vi "Create Live Random Data Tag Array.vi"() -> ()   [LabVIEW 2014]
uses:
  Tag.lvclass
  Anchor/Anchor.lvclass
panel:
  in  "Max h variatie":dbl=30.0 format="%#_13g"
  in  "Max V variatie":dbl=10.0 format="%#_13g"
  in  "DistanceLimitAnchor":dbl=150.0
  in  "Input AnchorArray":refnum<class "Anchor.lvclass">[](array[class])
  out "OutputArray":T1(array[cluster])
  in  "InputArray":T1(array[cluster])
  in  "TagsArray":refnum<class "Tag.lvclass">[](array[class])
  # "This VI creates a number of random data for each assigned tag in its array."
  # "tagID, X, Y, distances"
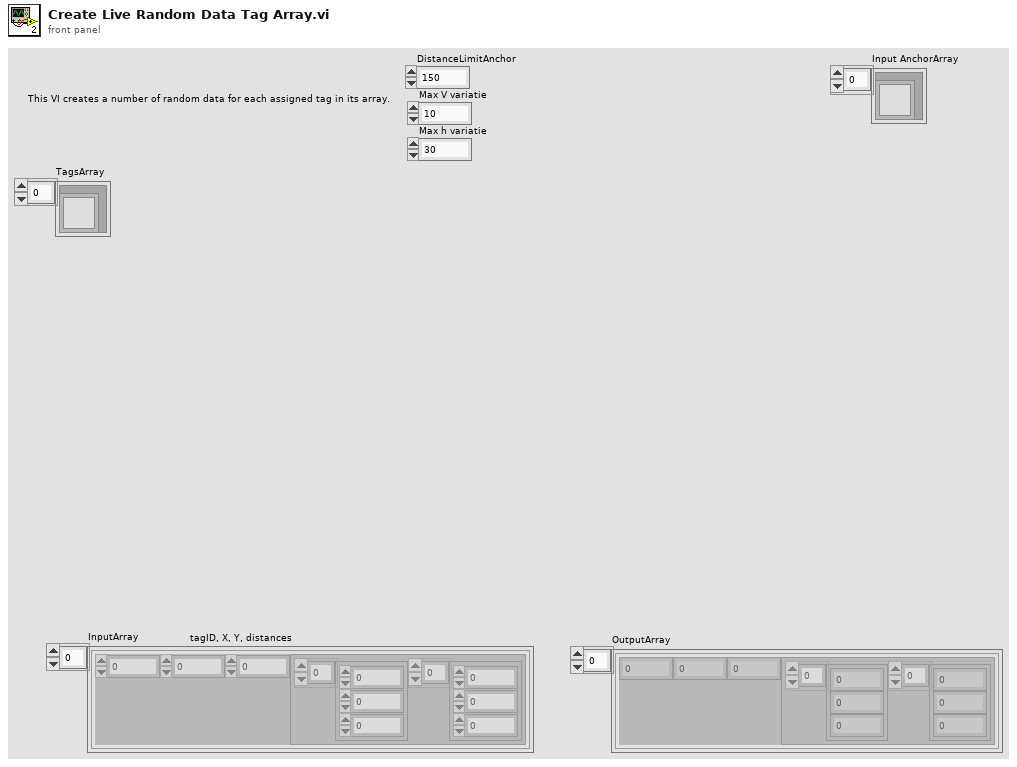
[diagram p1: front panel]
types:
  T1 = cluster{"Tag":dbl, "X":dbl, "Y":dbl, "AnchorIDDistanceCluster":cluster{"AnchorIDArray":dbl[], "AnchorDistancesArray":dbl[]}}[]
  T2 = cluster{"Tag.lvclass":refnum<class "Tag.lvclass">, "Intersections":cluster{"time [ms]":dbl, "x":dbl, "y":dbl, "Fout":bool, "Goed":bool}[]}[]
  T3 = cluster{"time [ms]":dbl, "x":dbl, "y":dbl, "Fout":bool, "Goed":bool}[]
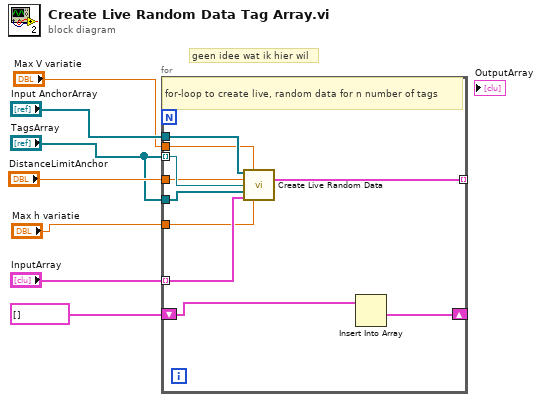
[diagram p0: block diagram]
diagram:
  # "geen idee wat ik hier wil"
  n1 = for {
    tunnel: "TagsArray" -> [w17] mode=indexing
    tunnel: "InputArray" -> [w15] mode=indexing
    tunnel: [w16] -> _ mode=indexing
    shift-right: [w14] -> _
    shift-left: T2 [] -> [w13]
    tunnel: "Input AnchorArray" -> [w12]
    tunnel: "DistanceLimitAnchor" -> [w11]
    tunnel: "TagsArray" -> [w10]
    tunnel: "Max V variatie" -> [w9]
    tunnel: "Max h variatie" -> [w8]
    # "for-loop to create live, random data for n number of tags"
    n2 = call "Create Live Random Data.vi"("Input AnchorArray"=w12, "Max V variatie"=w9, "DistanceLimitAnchor"=w11, "Tag.lvclass"=w17, "TagsArray"=w10, "Input"=w15, "Max h variatie"=w8) -> ("Intersections"=w16:T3)  [unwired: 5 in, 3 out]
    n3 = Insert Into Array(array=w13) -> (w14:T2)  [unwired: 2 in]
  }
